vi "spEVENTLOG Read Log.vi"(8 "error in (no error)":errorcluster) -> (0 "error out":errorcluster, 3 "Event Log Text":string)   [LabVIEW 2011]
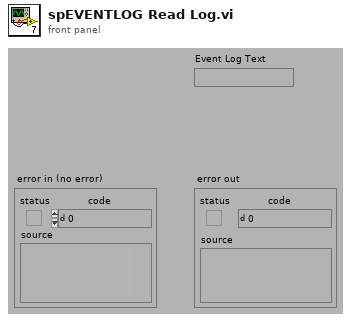
[diagram p1: front panel]
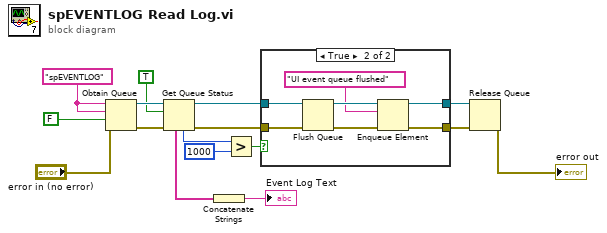
[diagram p0: block diagram]
diagram:
  w15 = "spEVENTLOG"
  n1 = Obtain Queue(name (unnamed)=w15, element data type=w15, create if not found? (T)=FALSE, error in (no error)="error in (no error)") -> (queue out=w13:refnum<queue>, error out=w12:errorcluster)  [unwired: 1 in, 1 out]
  n2 = Get Queue Status(queue=w13, return elements? (F)=TRUE, error in (no error)=w12) -> (queue out=w6:refnum<queue>, error out=w5:errorcluster, # elements in queue=w8:i32, elements=w10:string[])  [unwired: 4 out]
  n3 = Concatenate Strings(w10) -> (→"Event Log Text":string)
  n4 = Greater?(x=w8, y=1000) -> (0:w4:bool)
  n5 = case shown="True" w4 {
    tunnel: w6 -> [w18 w25]
    tunnel: w5 -> [w17 w24]
    tunnel: [w17 w20] -> w2
    tunnel: [w18 w19] -> w3
    frame False {
    }
    frame True {
      n6 = Flush Queue(queue=w25, error in (no error)=w24) -> (queue out=w23:refnum<queue>, error out=w21:errorcluster)  [unwired: 1 out]
      n7 = Enqueue Element(queue=w23, element="UI event queue flushed", error in (no error)=w21) -> (queue out=w19:refnum<queue>, error out=w20:errorcluster)  [unwired: 1 in, 1 out]
    }
  }
  n8 = Release Queue(queue=w3, error in (no error)=w2) -> (error out=→"error out":errorcluster)  [unwired: 1 in, 2 out]
